vi "enum_main.vi"() -> ()   [LabVIEW 2021]
panel:
  in  "Enum":enum16{"Team A", "Team B", "Team  D"}(ring)
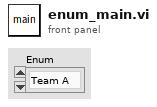
[diagram p1: front panel]
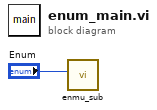
[diagram p0: block diagram]
diagram:
  n1 = call "enmu_sub.vi"("Enum"="Enum") -> ()  [unwired: 11 in]
